vi "Pulse Mode - Read Configurations.vi"   [LabVIEW 2014, in "Associated Power Technologies 8500 Series.lvlib"]
uses:
  <instrlib>/Associated Power Technologies 8500 Series/Associated Power Technologies 8500 Series.lvlib
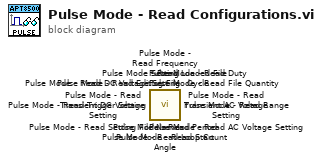
[diagram p0: block diagram]
diagram:
  n1 = call <instrlib>:"Pulse Mode - Read Period.vi"() -> ()  [unwired: 9 in, 3 out]
  n2 = call <instrlib>:"Pulse Mode - Read Duty Cycle.vi"() -> ()  [unwired: 9 in, 3 out]
  n3 = call <instrlib>:"Pulse Mode - Read Transient DC Voltage Setting.vi"() -> ()  [unwired: 9 in, 3 out]
  n4 = call <instrlib>:"Pulse Mode - Read Transient AC Voltage Setting.vi"() -> ()  [unwired: 9 in, 3 out]
  n5 = call <instrlib>:"Pulse Mode - Read Start Angle.vi"() -> ()  [unwired: 9 in, 3 out]
  n6 = call <instrlib>:"Pulse Mode - Read DC Voltage Setting.vi"() -> ()  [unwired: 9 in, 3 out]
  n7 = call <instrlib>:"Pulse Mode - Read Frequency Setting.vi"() -> ()  [unwired: 9 in, 3 out]
  n8 = call <instrlib>:"Pulse Mode - Read AC Voltage Setting.vi"() -> ()  [unwired: 9 in, 3 out]
  n9 = call <instrlib>:"Pulse Mode - Read Range.vi"() -> ()  [unwired: 9 in, 3 out]
  n10 = call <instrlib>:"Pulse Mode - Read Trigger Setting.vi"() -> ()  [unwired: 9 in, 3 out]
  n11 = call <instrlib>:"Pulse Mode - Read Loop Count.vi"() -> ()  [unwired: 9 in, 3 out]
  n12 = call <instrlib>:"Pulse Mode - Read Setting File Name.vi"() -> ()  [unwired: 9 in, 3 out]
  n13 = call <instrlib>:"Pulse Mode - Read File Quantity.vi"() -> ()  [unwired: 9 in, 3 out]
  n14 = call <instrlib>:"Pulse Mode - Read Loaded File.vi"() -> ()  [unwired: 9 in, 3 out]
  n15 = call <instrlib>:"Pulse Mode - Read Editing File.vi"() -> ()  [unwired: 9 in, 3 out]
